vi "Polarization Process Image.vi"(5 "imageOriginY_pixels":i32, 6 "sensorPolarPhase":i32(ring) items=["PolarPhase0", "PolarPhase45", "PolarPhase90", "PolarPhase135"], 7 "imageOriginX_pixels":i32, 8 "error in (no error)":errorcluster, 9 "Polarization Processing Type":T1, 10 "ImageData":refnum<k24>, 11 "PolarizationProcessor reference":refnum<k24>) -> (0 "error out":errorcluster, 2 "Output image data":dbl[][](array[numeric]), 3 "PolarizationProcessor reference out":refnum<k24>)   [LabVIEW 2019]
uses:
  Thor_Controls/Polarization Processing Type.ctl
  C:/code/ScientificCameraInterfaces/Installer/Scientific Camera Interfaces/LabVIEW/64_bit/Library_X64/Thorlabs.TSI.ImageDataInterfaces.dll
  code/ScientificCameraInterfaces/Installer/Scientific Camera Interfaces/LabVIEW/64_bit/Library_X64/Thorlabs.TSI.ImageDataInterfaces.dll
  C:/code/ScientificCameraInterfaces/Installer/Scientific Camera Interfaces/LabVIEW/64_bit/Library_X64/Thorlabs.TSI.PolarizationInterfaces.dll
  code/ScientificCameraInterfaces/Installer/Scientific Camera Interfaces/LabVIEW/64_bit/Library_X64/Thorlabs.TSI.PolarizationInterfaces.dll
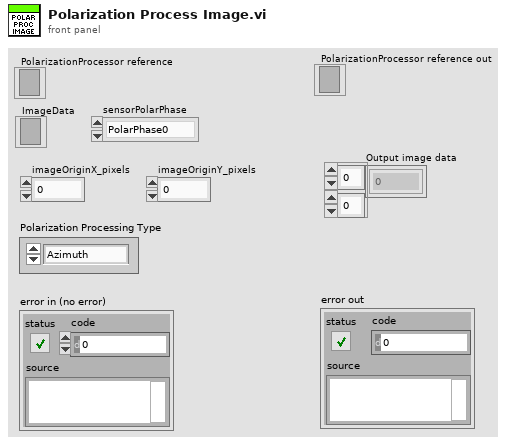
[diagram p1: front panel]
types:
  T1 = typedef "Polarization Processing Type.ctl" = enum16{"Azimuth", "DoLP", "Intensity"}
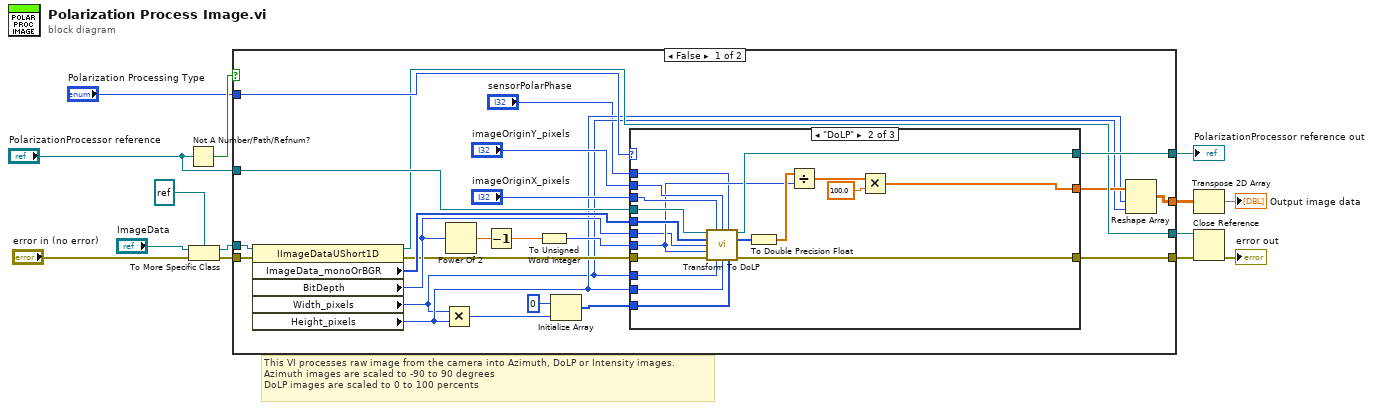
[diagram p0: block diagram]
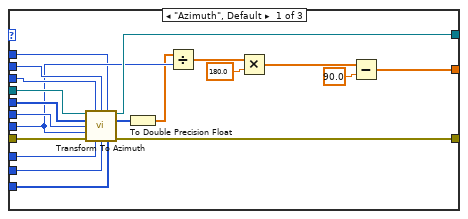
[diagram p2: hidden frame]
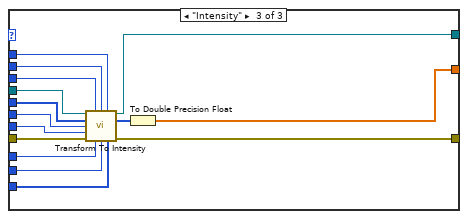
[diagram p3: hidden frame]
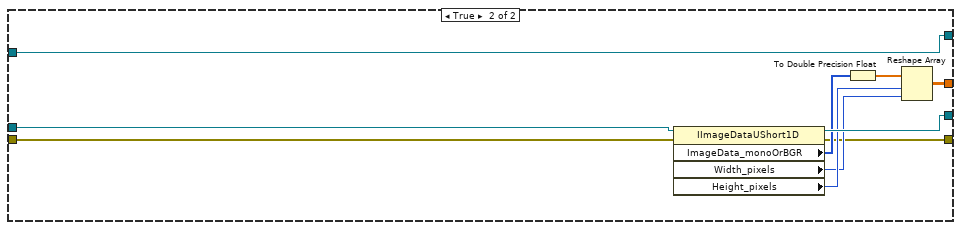
[diagram p4: hidden frame]
diagram:
  # "This VI processes raw image from the camera into Azimuth, DoLP or Intensity images.\nAzimuth images are scaled to -90 to 90 degrees\nDoLP images are scaled to 0 to 100 percents"
  n1 = Not A Number/Path/Refnum?(number/path/refnum="PolarizationProcessor reference") -> (NaN/Path/Refnum?=w14:bool)
  n2 = To More Specific Class(target class=refnum<k24> refnum, reference="ImageData", error in="error in (no error)") -> (specific class reference=w7:refnum<k24>, error out=w9:errorcluster)
  n3 = case shown="False" w14 {
    tunnel: "PolarizationProcessor reference" -> [w37 w100]
    tunnel: "Polarization Processing Type" -> [w24 _]
    tunnel: w7 -> [w36 w98]
    tunnel: w9 -> [w35 w99]
    tunnel: [w23 w100] -> w6
    tunnel: [w21 w91] -> w4
    tunnel: [w20 w97] -> w5
    tunnel: [w16 w92] -> w2
    frame False {
      n4 = property class="IImageDataUShort1D"(reference=w36, error in=w35) -> (reference out=w20:refnum<k24>, error out=w22:errorcluster, "ImageData_monoOrBGR"=w34:u16[], "BitDepth"=w29:i32, "Width_pixels"=w17:i32, "Height_pixels"=w18:i32)
      n5 = Multiply(x=w17, y=w18) -> (x*y=w32:i32)
      n6 = Power Of 2(x=w29) -> (2^x=w30:dbl)
      n7 = Decrement(x=w30) -> (x-1=w28:dbl)
      n8 = To Unsigned Word Integer(number=w28) -> (unsigned 16bit integer=w27:u16)
      n9 = Initialize Array(u16 0 ("element"), w32) -> (w31:u16[])
      n10 = case shown="\"DoLP\"" w24 {
        tunnel: w37 -> [w57 w75 w90]
        tunnel: w34 -> [w56 w74 w84]
        tunnel: w17 -> [w55 w73 w79]
        tunnel: w18 -> [w54 w72 w78]
        tunnel: w31 -> [w49 w63 w77]
        tunnel: w29 -> [w53 w59 w83]
        tunnel: w27 -> [w46 w60 w82]
        tunnel: "imageOriginX_pixels" -> [w52 w71 w80]
        tunnel: "imageOriginY_pixels" -> [w51 w70 w81]
        tunnel: [w50 w69 w87] -> w23
        tunnel: w22 -> [w48 w62 w89]
        tunnel: [w47 w68 w88] -> w21
        tunnel: [w39 w61 w85] -> w19
        tunnel: "sensorPolarPhase" -> [w38 w58 w76]
        frame "Azimuth", Default {
          n11 = call "Transform To Azimuth.vi"("PolarizationProcessor reference"=w57, "imageOriginX_pixels"=w52, "imageOriginY_pixels"=w51, "sensorPolarPhase"=w38, "inputImage"=w56, "inputImageBitDepth"=w53, "outputMaxValue"=w46, "error in (no error)"=w48, "imageWidth_pixels"=w55, "imageHeight_pixels"=w54, "Azimuth buffer input"=w49) -> ("PolarizationProcessor reference out"=w50:refnum<k24>, "Azimuth out"=w45:u16[], "error out"=w47:errorcluster)  [unwired: 2 in]
          n12 = To Double Precision Float(number=w45) -> (double precision float=w44:dbl[])
          n13 = Divide(x=w44, y=w46) -> (x/y=w43:dbl[])
          n14 = Multiply(x=w43, y=180.0) -> (x*y=w41:dbl[])
          n15 = Subtract(x=w41, y=90.0) -> (x-y=w39:dbl[])
        }
        frame "DoLP" {
          n16 = call "Transform To DoLP.vi"("PolarizationProcessor reference"=w75, "imageOriginX_pixels"=w71, "imageOriginY_pixels"=w70, "sensorPolarPhase"=w58, "inputImage"=w74, "inputImageBitDepth"=w59, "outputMaxValue"=w60, "error in (no error)"=w62, "imageWidth_pixels"=w73, "imageHeight_pixels"=w72, "DoLP buffer input"=w63) -> ("PolarizationProcessor reference out"=w69:refnum<k24>, "DoLP out"=w67:u16[], "error out"=w68:errorcluster)  [unwired: 2 in]
          n17 = To Double Precision Float(number=w67) -> (double precision float=w66:dbl[])
          n18 = Divide(x=w66, y=w60) -> (x/y=w65:dbl[])
          n19 = Multiply(x=w65, y=100.0) -> (x*y=w61:dbl[])
        }
        frame "Intensity" {
          n20 = call "Transform To Intensity.vi"("PolarizationProcessor reference"=w90, "imageOriginX_pixels"=w80, "imageOriginY_pixels"=w81, "sensorPolarPhase"=w76, "inputImage"=w84, "inputImageBitDepth"=w83, "outputMaxValue"=w82, "error in (no error)"=w89, "imageWidth_pixels"=w79, "imageHeight_pixels"=w78, "Intensity buffer input"=w77) -> ("PolarizationProcessor reference out"=w87:refnum<k24>, "Intensity out"=w86:u16[], "error out"=w88:errorcluster)  [unwired: 2 in]
          n21 = To Double Precision Float(number=w86) -> (double precision float=w85:dbl[])
        }
      }
      n22 = Reshape Array(w19, w18, w17) -> (w16:dbl[][])
    }
    frame True {
      n23 = property class="IImageDataUShort1D"(reference=w98, error in=w99) -> (reference out=w97:refnum<k24>, error out=w91:errorcluster, "ImageData_monoOrBGR"=w96:u16[], "Width_pixels"=w93:i32, "Height_pixels"=w94:i32)
      n24 = To Double Precision Float(number=w96) -> (double precision float=w95:dbl[])
      n25 = Reshape Array(w95, w94, w93) -> (w92:dbl[][])
    }
  }
  "PolarizationProcessor reference out" <- w6
  n26 = Transpose 2D Array(2D array=w2) -> (transposed array=→"Output image data":dbl[][])
  n27 = Close Reference(reference=w5, error in (no error)=w4) -> (error out=→"error out":errorcluster)
